vi "Disconnect.vi"(8 "error in (no error)":errorcluster, 11 "PXI-5441 in":refnum<class "PXI-5441.lvclass">) -> (0 "error out":errorcluster, 3 "PXI-5441 out":refnum<class "PXI-5441.lvclass">)   [LabVIEW 2023, in "PXI-5441.lvlib" / "PXI-5441.lvclass"]
uses:
  PXI-5441.lvclass
  PXI-5441.lvclass/PXI-5441.ctl
  IScope_interface/IStates_interface/IStates.lvclass
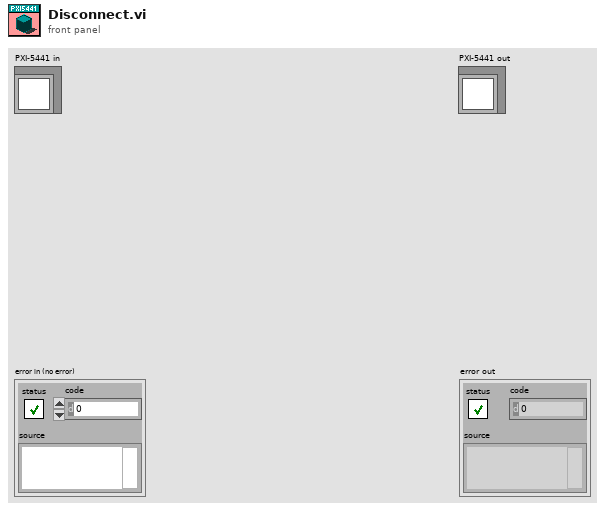
[diagram p1: front panel]
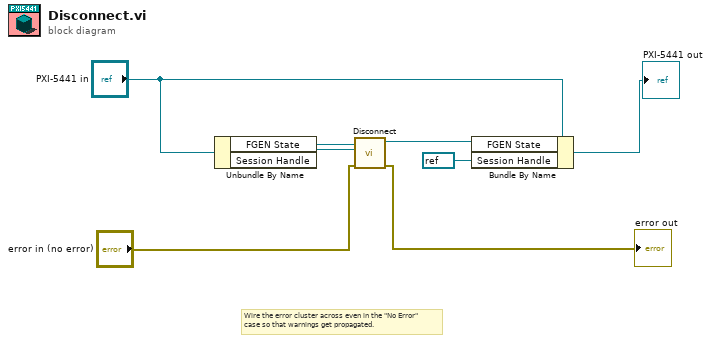
[diagram p0: block diagram]
diagram:
  # "Wire the error cluster across even in the \"No Error\"\ncase so that warnings get propagated."
  n1 = Unbundle By Name("PXI-5441 in") -> ("FGEN State"=w6:refnum<class "IStates.lvclass">, "Session Handle"=w3:refnum<k15>)
  n2 = call-dynamic "Disconnect.vi"("Error In"="error in (no error)", 10:w3, "object in"=w6) -> ("Error Out"=→"error out":errorcluster, "object out"=w5:refnum<class "IStates.lvclass">)  [unwired: 7 in]
  n3 = Bundle By Name(cluster="PXI-5441 in", "FGEN State"=w5, "Session Handle"=refnum<k15> refnum ("Resource Name")) -> (→"PXI-5441 out":refnum<class "PXI-5441.lvclass">)
